vi "catalog.wait_until_ingest_complete.vi"(6 "timeout (-1: never)":i32=-1, 8 "error in":errorcluster, 10 "datasetRid":string, 11 "Nominal Client":refnum<class "Nominal Client.lvclass">) -> (0 "error out":errorcluster, 3 "Nominal Client out":refnum<class "Nominal Client.lvclass">)   [LabVIEW 2020, in "Nominal Client.lvclass"]
doc: "Just for datasets"
uses:
  Nominal Client.lvclass
  Nominal Client.lvclass/Nominal Client.ctl
  catalog.get_ingest_progress_v2.vi
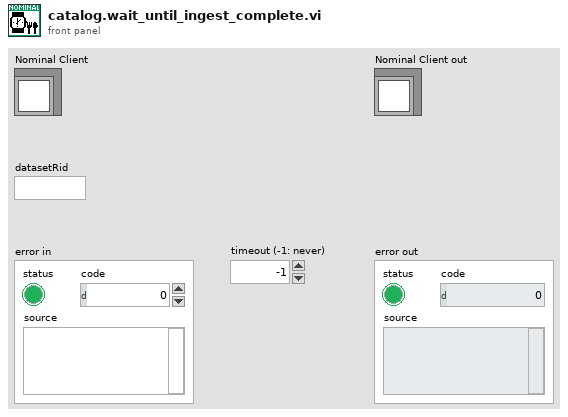
[diagram p1: front panel]
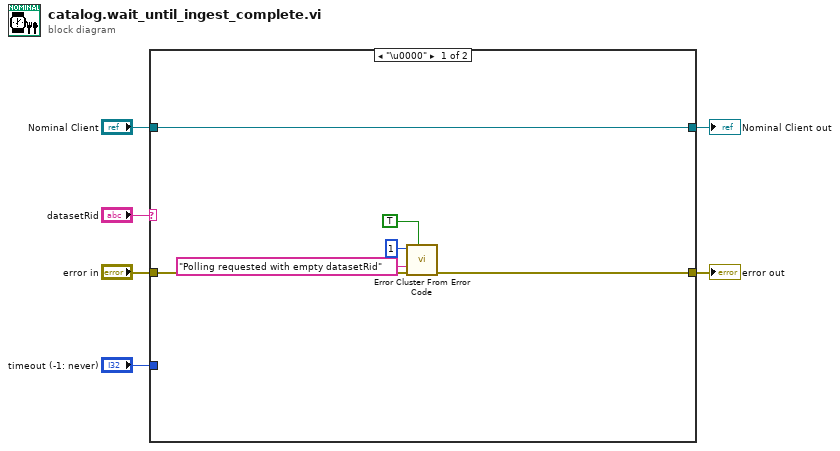
[diagram p0: block diagram]
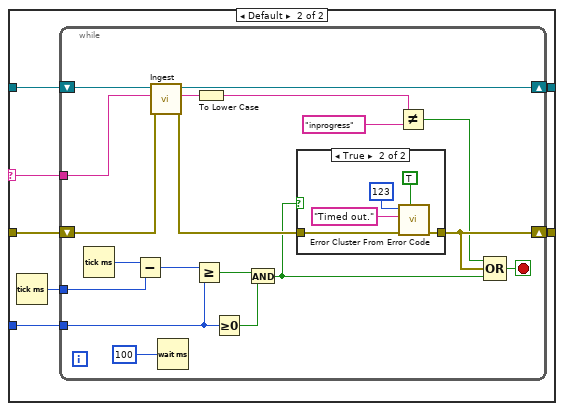
[diagram p2: hidden frame]
diagram:
  n1 = case shown="\"\"" "datasetRid" {
    selector: "datasetRid" -> [_ w13]
    tunnel: "Nominal Client" -> [w12 w19]
    tunnel: [w12 w18] -> w5
    tunnel: [w10 w17] -> w4
    tunnel: "error in" -> [w11 w16]
    tunnel: "timeout (-1: never)" -> [_ w14]
    frame "\u0000" {
      n2 = call <vilib>:"Error Cluster From Error Code.vi"("show call chain? (False)"=TRUE, "error in (no error)"=w11, "error message (\"\")"="Polling requested with empty datasetRid" ("error message (\"\")"), "error code (0)"=1) -> ("error out"=w10:errorcluster)  [unwired: 5 in]
    }
    frame Default {
      n3 = Tick Count (ms)() -> (millisecond timer value=w15:u32)
      n4 = while {
        shift-right: [w36] -> w18
        shift-left: w19 -> [w38]
        shift-right: [w24] -> w17
        shift-left: w16 -> [w37]
        tunnel: w15 -> [w32]
        tunnel: w14 -> [w30]
        tunnel: w13 -> [w20]
        stop <- w35 stop-if-true
        n5 = Tick Count (ms)() -> (millisecond timer value=w33:u32)
        n6 = Subtract(x=w33, y=w32) -> (x-y=w31:u32)
        n7 = call-poly "Ingest.vi"("error in"=w37, "datasetRid[]"=w20, "Nominal Client in"=w38) -> ("error out"=w23:errorcluster, "Status"=w27:string, "Nominal Client out"=w36:refnum<class "Nominal Client.lvclass">)  [unwired: 5 in, 1 out]
        n8 = Wait (ms)(milliseconds to wait=u32 100) -> ()  [unwired: 1 out]
        n9 = Greater Or Equal?(x=w31, y=w30) -> (x >= y?=w28:bool)
        n10 = To Lower Case(string=w27) -> (all lower case string=w26:string)
        n11 = Greater Or Equal To 0?(x=w30) -> (x >= 0?=w29:bool)
        n12 = And(x=w28, y=w29) -> (x .and. y?=w22:bool)
        n13 = case shown="True" w22 {
          tunnel: [w39 w41] -> w24
          tunnel: w23 -> [w39 w40]
          frame False {
          }
          frame True {
            n14 = call <vilib>:"Error Cluster From Error Code.vi"("show call chain? (False)"=TRUE, "error in (no error)"=w40, "error message (\"\")"="Timed out." ("error message (\"\")"), "error code (0)"=123) -> ("error out"=w41:errorcluster)  [unwired: 5 in]
          }
        }
        n15 = Not Equal?(x=w26, y="inprogress") -> (x != y?=w21:bool)
        n16 = Compound Arithmetic op=OR(w21, w24, w22) -> (w35:bool)
      }
    }
  }
  "Nominal Client out" <- w5
  "error out" <- w4
